vi "Rectangle Comparison.vi"(6 "Line Border":cluster{"Top":dbl, "Bottom":dbl}={"Top"=6.0, "Bottom"=1.0}, 9 "Second":dbl[](array[numeric]), 11 "First":dbl[](array[numeric])) -> (0 "Rect":T1, 1 "Line":T1, 3 "Scores":T2)   [LabVIEW 2016]
panel:
  # "This vi has been modified by team 1726 \nin order to process the vertical stripes \nlocated at the lift station. D.T. 1/115/17"
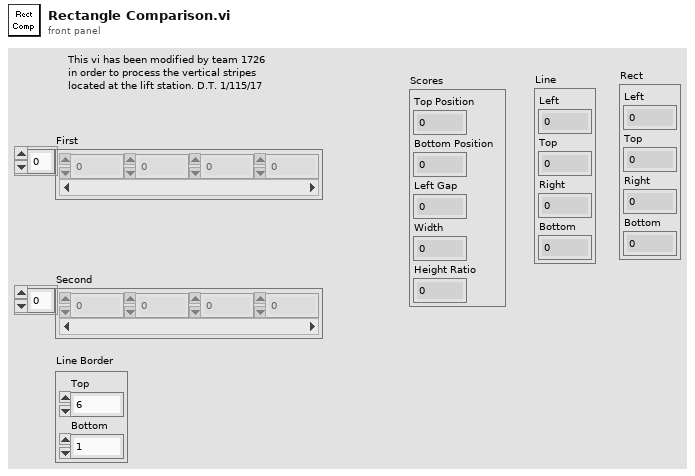
[diagram p1: front panel]
types:
  T1 = cluster{"Left":dbl, "Top":dbl, "Right":dbl, "Bottom":dbl}
  T2 = cluster{"Top Position":dbl, "Bottom Position":dbl, "Left Gap":dbl, "Width":dbl, "Height Ratio":dbl}
  T3 = cluster{"[0]":dbl, "[1]":dbl, "[2]":dbl, "[3]":dbl}
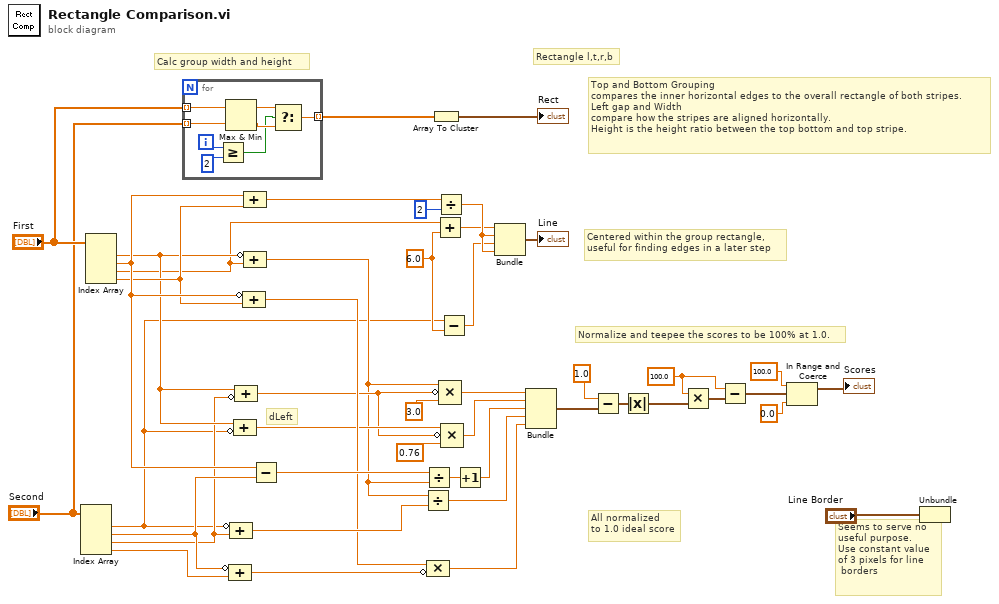
[diagram p0: block diagram]
diagram:
  w4 = 6.0 ("y")
  w28 = 100.0 ("x/y")
  # "Seems to serve no\nuseful purpose.\nUse constant value \nof 3 pixels for line\n borders"
  # "dLeft"
  # "Centered within the group rectangle,\nuseful for finding edges in a later step"
  # "All normalized\nto 1.0 ideal score"
  # "Normalize and teepee the scores to be 100% at 1.0."
  # "Top and Bottom Grouping\ncompares the inner horizontal edges to the overall rectangle of both stripes.\nLeft gap and Width\ncompare how the stripes are aligned horizontally.\nHeight is the height ratio between the top bottom and top stripe."
  # "Calc group width and height"
  # "Rectangle l,t,r,b"
  n1 = Index Array(array="Second") -> (element #1=w1:dbl, element #2=w12:dbl, element #3=w8:dbl, element #4=w20:dbl)  [unwired: 4 in]
  n2 = Index Array(array="First") -> (element #1=w9:dbl, element #2=w11:dbl, element #3=w2:dbl, element #4=w10:dbl)  [unwired: 4 in]
  n3 = for {
    tunnel: "First" -> [w53] mode=indexing
    tunnel: "Second" -> [w52] mode=indexing
    tunnel: [w46] -> w33 mode=indexing
    i -> [w50]
    n4 = Greater Or Equal?(x=w50, y=2) -> (x >= y?=w47:bool)
    n5 = Max & Min(x=w53, y=w52) -> (max(x,y)=w49:dbl, min(x,y)=w48:dbl)
    n6 = Select(t=w49, s=w47, f=w48) -> (s? t:f=w46:dbl)
  }
  n7 = Compound Arithmetic op=ADD(invert w12, w20) -> (w44:dbl)
  n8 = Compound Arithmetic op=ADD(invert w1, w8) -> (w45:dbl)
  n9 = Compound Arithmetic op=ADD(w9, invert w1) -> (w18:dbl)
  n10 = Compound Arithmetic op=ADD(w9, invert w8) -> (w17:dbl)
  n11 = Compound Arithmetic op=ADD(invert w11, w10) -> (w19:dbl)
  n12 = Compound Arithmetic op=ADD(w11, w10) -> (w38:dbl)
  n13 = Compound Arithmetic op=ADD(invert w9, w2) -> (w3:dbl)
  n14 = Subtract(x=w11, y=w12) -> (x-y=w43:dbl)
  n15 = Divide(x=w3, y=w45) -> (x/y=w41:dbl)
  n16 = Divide(x=w43, y=w3) -> (x/y=w39:dbl)
  n17 = Compound Arithmetic op=MULTIPLY(w19, invert w44) -> (w40:dbl)
  n18 = Array To Cluster(array=w33) -> (cluster=→"Rect":T3)
  n19 = Add(x=w2, y=w4) -> (x+y=w6:dbl)
  n20 = Divide(x=w38, y=2) -> (x/y=w7:dbl)
  n21 = Subtract(x=w1, y=w4) -> (x-y=w5:dbl)
  n22 = Compound Arithmetic op=MULTIPLY(w3, invert w17, 3.0 ("y")) -> (w42:dbl)
  n23 = Compound Arithmetic op=MULTIPLY(w18, invert w17, 0.76 ("y")) -> (w16:dbl)
  n24 = Increment(x=w39) -> (x+1=w31:dbl)
  n25 = Bundle(w6, w7, w5, w7) -> (→"Line":cluster{dbl, dbl, dbl, dbl})  [unwired: 1 in]
  n26 = Bundle(w42, w16, w31, w41, w40) -> (w22:cluster{dbl, dbl, dbl, dbl, dbl})  [unwired: 1 in]
  n27 = Subtract(x=1.0 ("y"), y=w22) -> (x-y=w26:cluster{dbl, dbl, dbl, dbl, dbl})
  n28 = Absolute Value(x=w26) -> (abs(x)=w29:cluster{dbl, dbl, dbl, dbl, dbl})
  n29 = Multiply(x=w28, y=w29) -> (x*y=w30:cluster{dbl, dbl, dbl, dbl, dbl})
  n30 = Subtract(x=w28, y=w30) -> (x-y=w25:cluster{dbl, dbl, dbl, dbl, dbl})
  n31 = In Range and Coerce(upper limit=100.0, x=w25, lower limit=0.0) -> (coerced(x)=→"Scores":cluster{dbl, dbl, dbl, dbl, dbl})  [unwired: 1 out]
  n32 = Unbundle("Line Border") -> ()  [unwired: 2 out]
